vi "receiveEvent.vi"(8 "error in (no error)":errorcluster, 10 "data":refnum<class>, 11 "ExperimentControlEvents in":refnum<class "ExperimentControlEvents.lvclass">) -> (0 "error out":errorcluster, 2 "Enum":T1(ring), 3 "ExperimentControlEvents out":refnum<class "ExperimentControlEvents.lvclass">)   [LabVIEW 2011, in "Views.lvlib" / "ExperimentControl.lvlib" / "ExperimentControlEvents.lvclass"]
uses:
  ExperimentControlEvents.lvclass
  ExperimentControlEvents.lvclass/ExperimentControlEvents.ctl
  Events/Event.lvclass
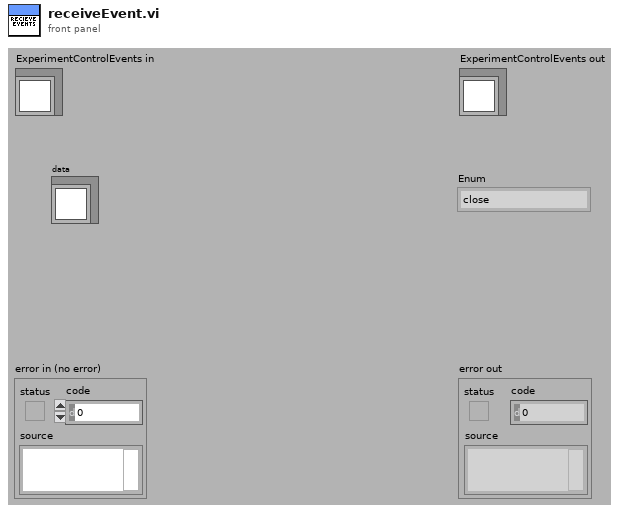
[diagram p1: front panel]
types:
  T1 = enum16{"close", "stopRunning", "runSingleScript", "runExperiment", "runExperimentScript", "Unregistered", "hasStopped"}
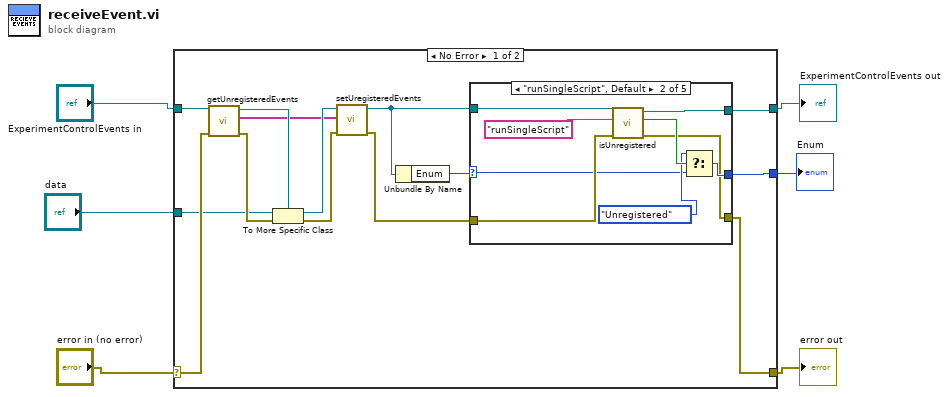
[diagram p0: block diagram]
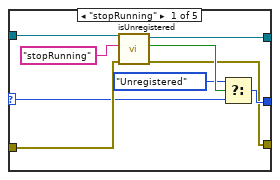
[diagram p2: hidden frame]
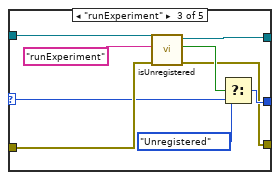
[diagram p3: hidden frame]
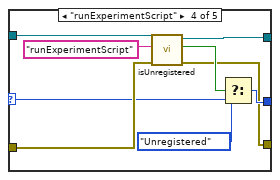
[diagram p4: hidden frame]
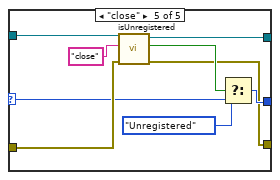
[diagram p5: hidden frame]
diagram:
  n1 = case shown="No Error" "error in (no error)" {
    selector: "error in (no error)" -> [w8 w67]
    tunnel: [w18 w67] -> w3
    tunnel: [w20 w66] -> w5
    tunnel: "ExperimentControlEvents in" -> [w16 w66]
    tunnel: "data" -> [w7 _]
    tunnel: [w19 _] -> w1
    frame No Error {
      n2 = call "getUnregisteredEvents.vi"("error in (no error)"=w8, "Event.lvclass in"=w16) -> ("error out"=w9:errorcluster, "unregisteredEvents"=w13:string[], "Event.lvclass out"=w15:refnum<class "ExperimentControlEvents.lvclass">)  [unwired: 7 in]
      n3 = To More Specific Class(target class=w15, reference=w7, error in=w9) -> (specific class reference=w14:refnum<class "ExperimentControlEvents.lvclass">, error out=w11:errorcluster)
      n4 = call "setUregisteredEvents.vi"("error in (no error)"=w11, "unregisteredEvents"=w13, "Event.lvclass in"=w14) -> ("error out"=w10:errorcluster, "Event.lvclass out"=w12:refnum<class "ExperimentControlEvents.lvclass">)  [unwired: 7 in]
      n5 = Unbundle By Name(w12) -> ("Enum"=w17:T1)
      n6 = case shown="\"runSingleScript\", Default" w17 {
        selector: w17 -> [w23 w32 w41 w50 w59]
        tunnel: w12 -> [w29 w38 w47 w56 w65]
        tunnel: [w28 w37 w46 w55 w64] -> w20
        tunnel: w10 -> [w26 w35 w44 w53 w62]
        tunnel: [w22 w31 w40 w49 w58] -> w19
        tunnel: [w21 w30 w39 w48 w57] -> w18
        frame "stopRunning" {
          n7 = call "isUnregistered.vi"("error in (no error)"=w26, "name"="stopRunning", "Event in"=w29) -> ("error out"=w21:errorcluster, "unregistered"=w25:bool, "Event out"=w28:refnum<class "ExperimentControlEvents.lvclass">)  [unwired: 6 in]
          n8 = Select(t=enum16{"Open", "Save", "Close", "Unregistered"}."Unregistered" ("Enum"), s=w25, f=w23) -> (s? t:f=w22:u16)
        }
        frame "runSingleScript", Default {
          n9 = call "isUnregistered.vi"("error in (no error)"=w35, "name"="runSingleScript", "Event in"=w38) -> ("error out"=w30:errorcluster, "unregistered"=w34:bool, "Event out"=w37:refnum<class "ExperimentControlEvents.lvclass">)  [unwired: 6 in]
          n10 = Select(t=enum16{"Open", "Save", "Close", "Unregistered"}."Unregistered" ("Enum"), s=w34, f=w32) -> (s? t:f=w31:u16)
        }
        frame "runExperiment" {
          n11 = call "isUnregistered.vi"("error in (no error)"=w44, "name"="runExperiment", "Event in"=w47) -> ("error out"=w39:errorcluster, "unregistered"=w43:bool, "Event out"=w46:refnum<class "ExperimentControlEvents.lvclass">)  [unwired: 6 in]
          n12 = Select(t=enum16{"Open", "Save", "Close", "Unregistered"}."Unregistered" ("Enum"), s=w43, f=w41) -> (s? t:f=w40:u16)
        }
        frame "runExperimentScript" {
          n13 = call "isUnregistered.vi"("error in (no error)"=w53, "name"="runExperimentScript", "Event in"=w56) -> ("error out"=w48:errorcluster, "unregistered"=w52:bool, "Event out"=w55:refnum<class "ExperimentControlEvents.lvclass">)  [unwired: 6 in]
          n14 = Select(t=enum16{"Open", "Save", "Close", "Unregistered"}."Unregistered" ("Enum"), s=w52, f=w50) -> (s? t:f=w49:u16)
        }
        frame "close" {
          n15 = call "isUnregistered.vi"("error in (no error)"=w62, "name"="close", "Event in"=w65) -> ("error out"=w57:errorcluster, "unregistered"=w61:bool, "Event out"=w64:refnum<class "ExperimentControlEvents.lvclass">)  [unwired: 6 in]
          n16 = Select(t=enum16{"Open", "Save", "Close", "Unregistered"}."Unregistered" ("Enum"), s=w61, f=w59) -> (s? t:f=w58:u16)
        }
      }
    }
    frame Error {
    }
  }
  "error out" <- w3
  "ExperimentControlEvents out" <- w5
  "Enum" <- w1
